vi "Parse Raw Data Into Subsystems.vi"(1 "Table In":string[][](table), 5 "Error In":errorcluster, 7 "SSC Column":i32) -> (15 "Tables Out":string[][][](array[string]), 17 "SSC Names":string[](array[string]), 19 "Error Out":errorcluster)   [LabVIEW 2020]
uses:
  c268785e-82ed-4add-a62a-025e663894ef.vi
  7712e8bb-2786-4653-b74e-fc17249f03f2.vi
  <vilib>/Array/Sort 2D Array - Pop Stack.vi
  <vilib>/Array/Sort 2D Array - Push Stack.vi
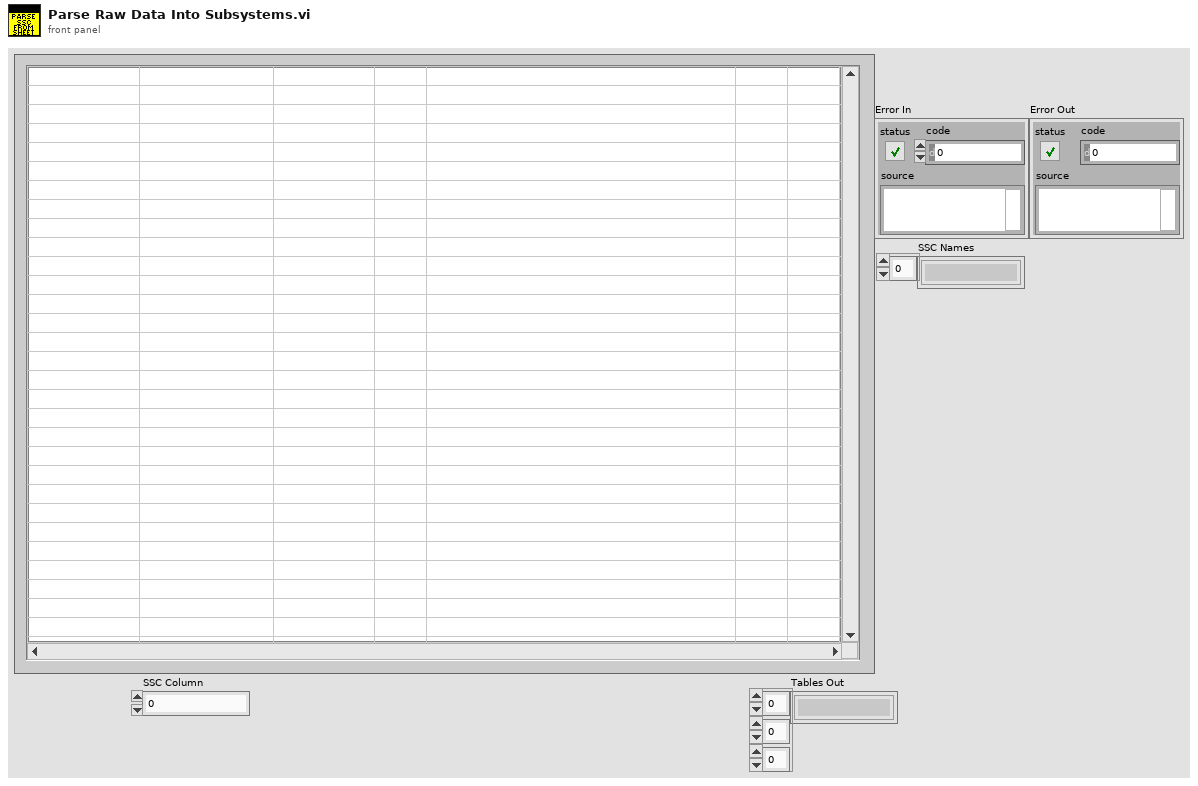
[diagram p1: front panel]
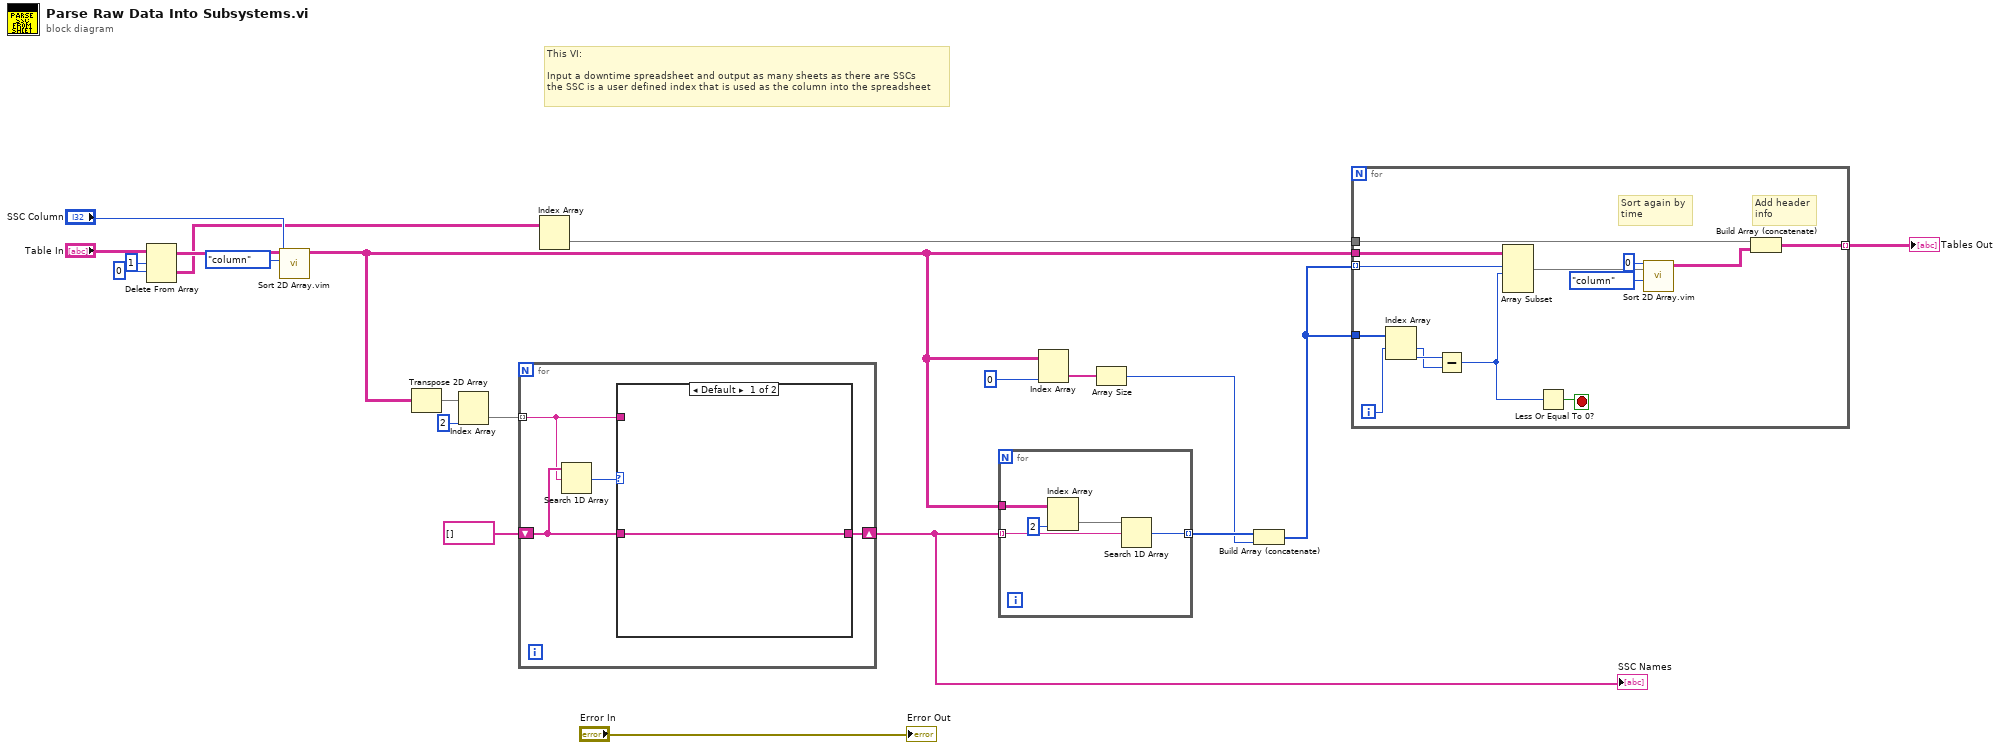
[diagram p0: block diagram]
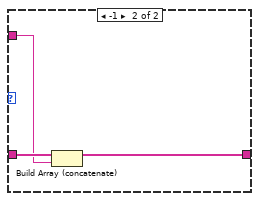
[diagram p2: hidden frame]
diagram:
  # "This VI:\n\nInput a downtime spreadsheet and output as many sheets as there are SSCs\nthe SSC is a user defined index that is used as the column into the spreadsheet"
  n1 = Delete From Array(array="Table In", length=1, index (row)=0) -> (deleted portion=w2:string[][], array with subset deleted=w15:string[][])  [unwired: 1 in]
  n2 = call "Sort 2D Array.vim"("index"="SSC Column", "dimension to index (column)"=enum16{"column", "row"}."column", "2D array"=w15) -> ("sorted 2D array"=w10:string[][])  [unwired: 7 in, 1 out]
  n3 = Transpose 2D Array(2D array=w10) -> (transposed array=w21:string[][])
  n4 = Index Array(array=w21, index (row)=2) -> (element=w19:string[])  [unwired: 1 in]
  n5 = for {
    tunnel: w19 -> [w22] mode=indexing
    shift-right: [w23] -> w16
    shift-left: string[] [] -> [w24]
    n6 = Search 1D Array(1D array=w24, element=w22) -> (index of element=w25:i32)  [unwired: 1 in]
    n7 = case shown="Default" w25 {
      tunnel: w22 -> [_ w27]
      tunnel: [w26 w28] -> w23
      tunnel: w24 -> [w26 w29]
      frame Default {
      }
      frame -1 {
        n8 = Build Array (concatenate)(w29, w27) -> (w28:string[])
      }
    }
  }
  "SSC Names" <- w16
  n9 = Index Array(array=w2) -> (element=w1:string[])  [unwired: 2 in]
  n10 = for {
    tunnel: w10 -> [w34]
    tunnel: w16 -> [w30] mode=indexing
    tunnel: [w31] -> w12 mode=indexing
    n11 = Index Array(array=w34, index (col)=2 ("disabled index (col)")) -> (element=w32:string[])  [unwired: 1 in]
    n12 = Search 1D Array(1D array=w32, element=w30) -> (index of element=w31:i32)  [unwired: 1 in]
  }
  n13 = Index Array(array=w10, index (col)=0 ("disabled index (col)")) -> (element=w8:string[])  [unwired: 1 in]
  n14 = Array Size(array=w8) -> (size(s)=w7:i32)
  n15 = Build Array (concatenate)(w12, w7) -> (w11:i32[])
  n16 = for {
    tunnel: w10 -> [w47]
    tunnel: w11 -> [w48] mode=indexing
    tunnel: [w36] -> w6 mode=indexing
    tunnel: w11 -> [w46]
    tunnel: w1 -> [w35]
    i -> [w43]
    stop <- w41 stop-if-true
    # "Add header\ninfo"
    # "Sort again by \ntime"
    n17 = Index Array(array=w46, index #1=w43) -> (element #1=w44:i32, element #2=w45:i32)  [unwired: 1 in]
    n18 = Subtract(x=w45, y=w44) -> (x-y=w42:i32)
    n19 = Array Subset(array=w47, index (row)=w48, length (row)=w42) -> (w38:string[][])  [unwired: 2 in]
    n20 = Less Or Equal To 0?(x=w42) -> (x <= 0?=w41:bool)
    n21 = call "Sort 2D Array.vim"("index"=0, "dimension to index (column)"=enum16{"column", "row"}."column", "2D array"=w38) -> ("sorted 2D array"=w37:string[][])  [unwired: 7 in, 1 out]
    n22 = Build Array (concatenate)(w35, w37) -> (w36:string[][])
  }
  "Tables Out" <- w6
  "Error Out" <- "Error In"
